vi "GetAttributeByName.vi"(8 "error in (no error)":errorcluster, 10 "AttrName":string, 11 "SMO in":refnum<class "SMO.lvclass">) -> (0 "error out":errorcluster, 1 "found":bool, 2 "Attribute":refnum<class "Attribute.lvclass">, 3 "SMO out":refnum<class "SMO.lvclass">)   [LabVIEW 2013, in "SMO.lvclass"]
uses:
  SMO.lvclass
  Support/Attribute/Attribute.lvclass
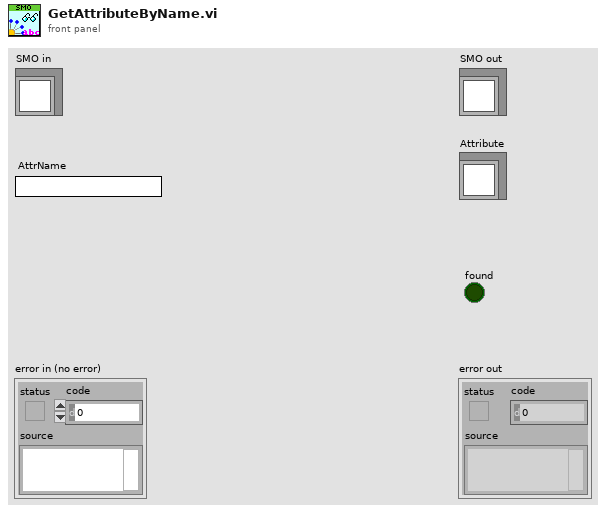
[diagram p1: front panel]
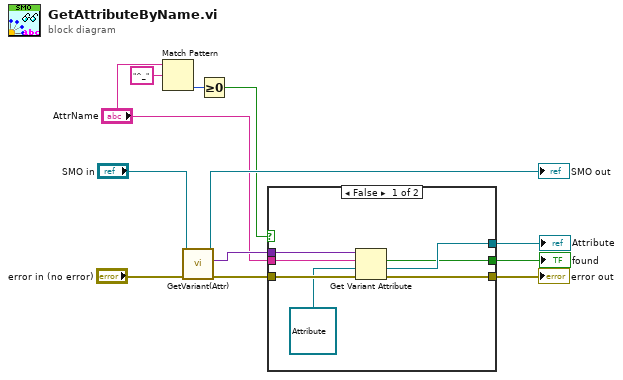
[diagram p0: block diagram]
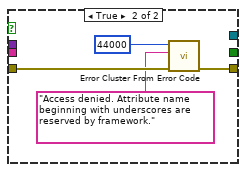
[diagram p2: hidden frame]
diagram:
  n1 = Match Pattern(string="AttrName", regular expression="^_") -> (offset past match=w2:i32)  [unwired: 1 in, 3 out]
  n2 = call "GetVariant(Attr).vi"("error in (no error)"="error in (no error)", "SMO in"="SMO in") -> ("error out"=w9:errorcluster, "[Attributes]"=w7:variant, "SMO out"=→"SMO out":refnum<class "SMO.lvclass">)  [unwired: 7 in]
  n3 = Greater Or Equal To 0?(x=w2) -> (x >= 0?=w1:bool)
  n4 = case shown="False" w1 {
    tunnel: w9 -> [w19 w22]
    tunnel: [w18 w23] -> w8
    tunnel: w7 -> [w16 _]
    tunnel: [w15 _] -> w6
    tunnel: [w14 _] -> w5
    tunnel: "AttrName" -> [w13 _]
    frame False {
      n5 = Get Variant Attribute(Variant=w16, name=w13, default value (empty Variant)=refnum<class "Attribute.lvclass"> refnum ("Attribute.lvclass"), error in=w19) -> (found=w14:bool, value=w15:refnum<class "Attribute.lvclass">, error out=w18:errorcluster)  [unwired: 1 out]
    }
    frame True {
      n6 = call <vilib>:"Error Cluster From Error Code.vi"("error in (no error)"=w22, "error message (\"\")"="Access denied. Attribute name beginning with underscores are reserved by framework." ("error message (\"\")"), "error code (0)"=44000) -> ("error out"=w23:errorcluster)  [unwired: 6 in]
    }
  }
  "error out" <- w8
  "Attribute" <- w6
  "found" <- w5
